vi "merFISH_set_autofocus_on_track.vi"(5 "queue ASI stage":refnum<queue>, 6 "error in":errorcluster, 7 "Slope":dbl, 8 "QPD ref":T1, 9 "queue piezo":refnum<queue>) -> (0 "error out":errorcluster)   [LabVIEW 2015]
uses:
  CONTROLS/Q_MCL_piezo_element.ctl
  CONTROLS/Q_ASI_stage_element.ctl
  <vilib>/Analysis/_algsub.llb/Vector Norm Type.ctl
  <vilib>/Analysis/_algsub.llb/Real Vector Norm.vi
  GLOBAL/Global_MCL_piezo.vi
  GLOBAL/Global_MAIN.vi
  GLOBAL/Global_FPGA.vi
  GLOBAL/Global_ABORT.vi
  <vilib>/regexp/Match Regular Expression.xnode
  <vilib>/Analysis/NI_AALPro.lvlib
panel:
  in  "abort":bool
  out "setpoint found":bool
  in  "resume":bool
  out "norm":dbl
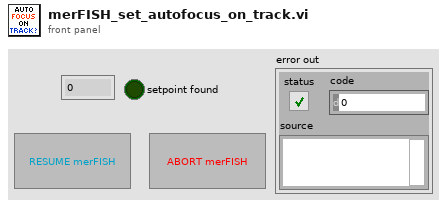
[diagram p1: front panel]
types:
  T1 = cluster{"X":sgl, "Y":sgl, "SUM":sgl, "count":u32}
  T2 = typedef "Q_MCL_piezo_element.ctl" = cluster{"variant":variant, "Instruction":enum16{"Piezo_idle", "Piezo_initialize", "Piezo_error", "Piezo_security_stop", "Piezo_read_z", "Piezo_move_z", "Piezo_keyboard_move", "Piezo_close_autofocus_calibration_ramp", "Piezo_change_init_state", "Piezo_init_autofocus", "Piezo_init_autofocus_merFISH_TL", "Piezo_autofocus", "Piezo_autofocus_merFISH_TL", "Piezo_stop_autofocus", "Piezo_stop_autofocus_merFISH_TL", "Piezo_autofocus_lost", "Piezo_resume_autofocus_merFISH_TL", "Piezo_check_z_position_merFISH_TL", "Piezo_init_ramp", "Piezo_move_z_ramp", "Piezo_close_ramp", "Piezo_close_merFISH", "Piezo_stop"}}
  T3 = typedef "NI_AALPro.lvlib/Vector Norm Type.ctl" = u16
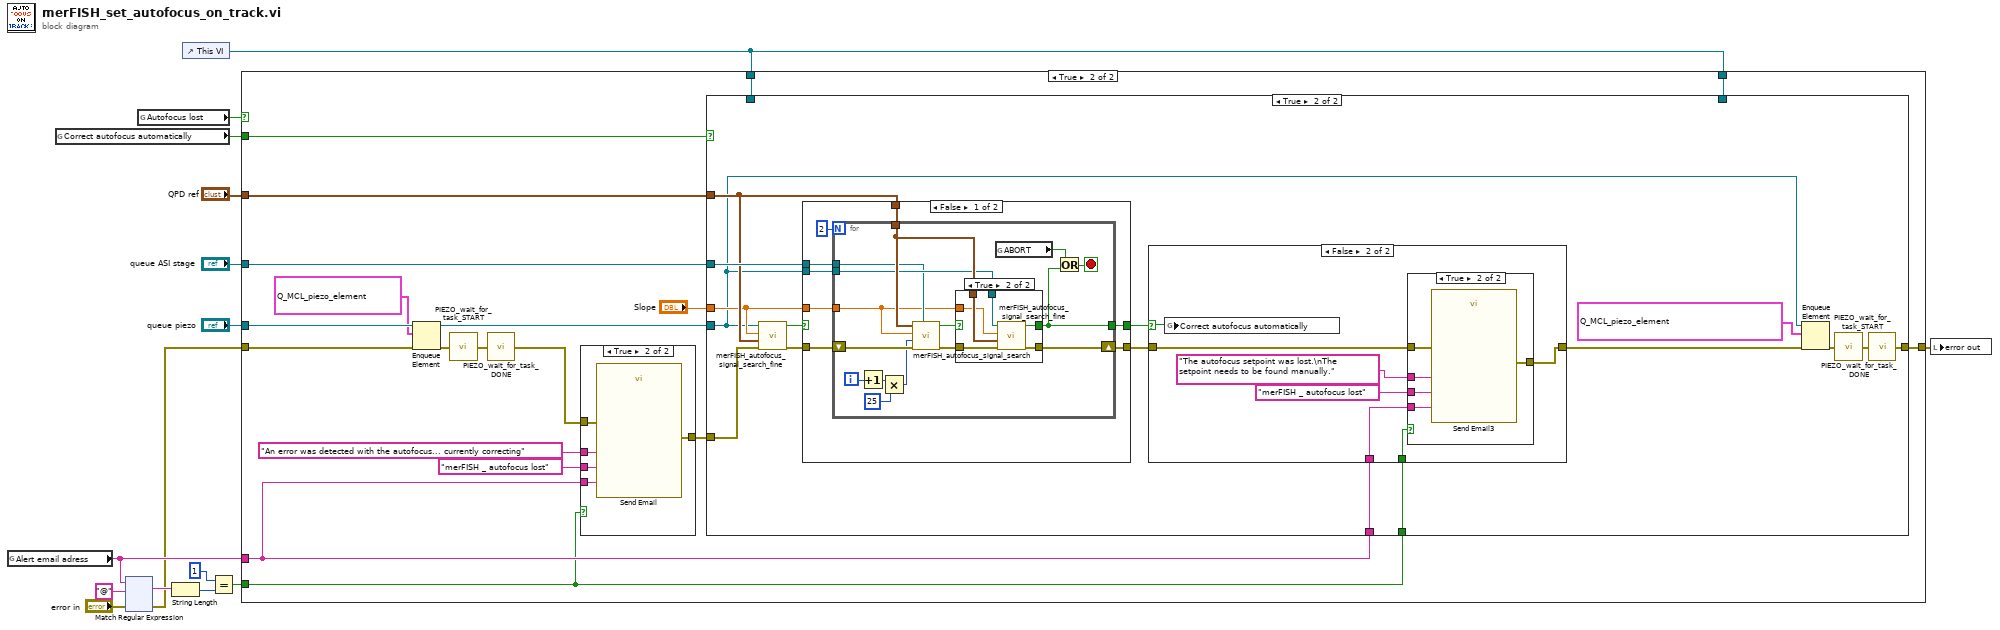
[diagram p0: block diagram]
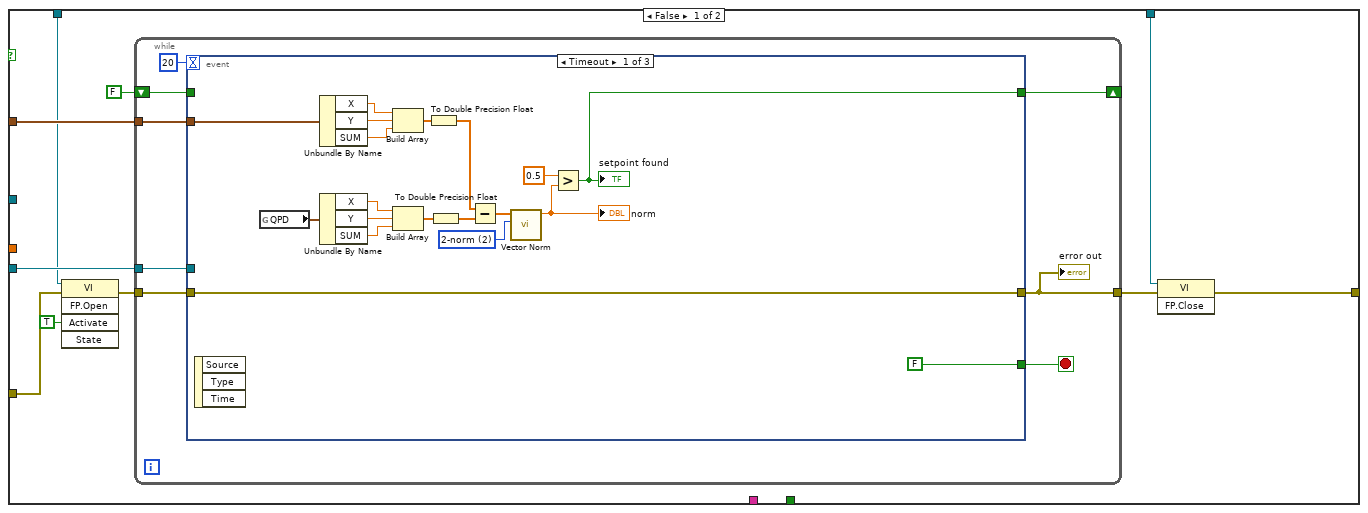
[diagram p4: hidden frame]
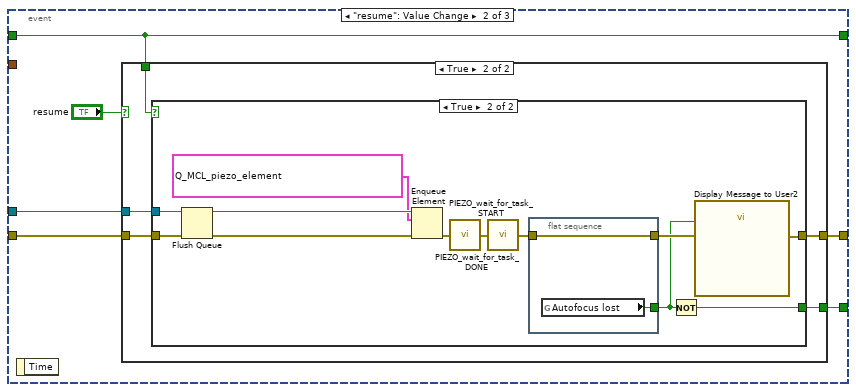
[diagram p5: hidden frame]
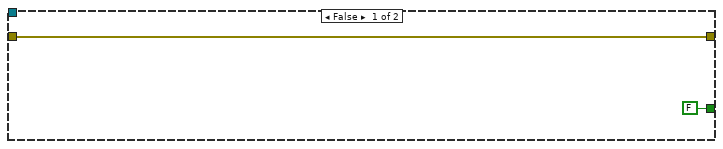
[diagram p6: hidden frame]
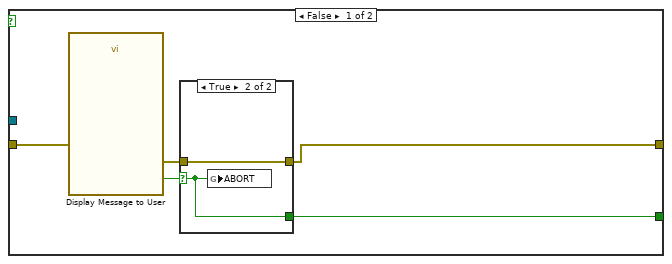
[diagram p7: hidden frame]
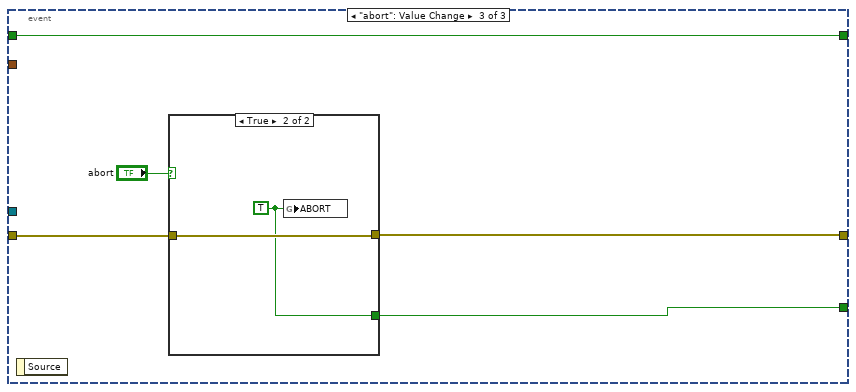
[diagram p9: hidden frame]
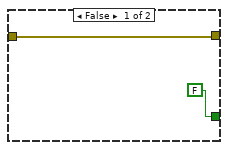
[diagram p10: hidden frame]
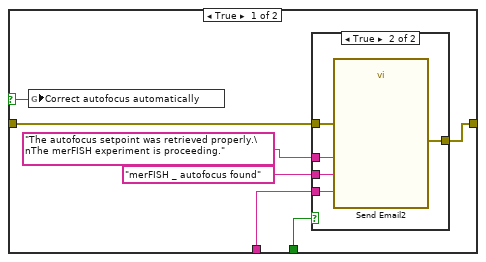
[diagram p13: hidden frame]
diagram:
  n1 = global read "Global_MAIN.vi" "Alert email adress"() -> (w5:string)
  n2 = global read "Global_MAIN.vi" "Correct autofocus automatically"() -> (w12:bool)
  n3 = xnode "Match Regular Expression"("input string"=w5, "regular expression"="@", "error in"="error in") -> ("whole match"=w7:string, "error out"=w3:errorcluster)  [unwired: 3 in, 3 out]
  n4 = global read "Global_MCL_piezo.vi" "Autofocus lost"() -> (w15:bool)
  n5 = String Length(string=w7) -> (length=w8:i32)
  n6 = control-ref of="This VI"() -> (w10:refnum<vi>)
  n7 = Equal?(x=1 ("y"), y=w8) -> (x = y?=w1:bool)
  n8 = case shown="True" w15 {
    tunnel: w3 -> [w16 w18]
    tunnel: "QPD ref" -> [_ w35]
    tunnel: "queue piezo" -> [_ w31]
    tunnel: [w16 w21] -> w13
    tunnel: w10 -> [_ w22]
    tunnel: w12 -> [_ w29]
    tunnel: "queue ASI stage" -> [_ w28]
    tunnel: w10 -> [_ w23]
    tunnel: w5 -> [_ w20]
    tunnel: w1 -> [_ w17]
    frame False {
    }
    frame True {
      n9 = Enqueue Element(queue=w31, element=T2 {"variant"=variant, "Instruction"=enum."Piezo_autofocus_lost"}, error in (no error)=w18) -> (queue out=w33:refnum<queue>, error out=w34:errorcluster)  [unwired: 1 in, 1 out]
      n10 = call "PIEZO_wait_for_task_START.vi"("error in"=w34) -> ("error out"=w32:errorcluster)
      n11 = call "PIEZO_wait_for_task_DONE.vi"("error in"=w32) -> ("error out"=w27:errorcluster)
      n12 = case shown="True" w17 {
        tunnel: w27 -> [w36 w41]
        tunnel: [w36 w40] -> w26
        tunnel: "merFISH _ autofocus lost" ("Subject") -> [_ w39]
        tunnel: "An error was detected with the autofocus... currently correcting" ("Message") -> [_ w38]
        tunnel: w20 -> [_ w37]
        frame False {
        }
        frame True {
          n13 = call "Send Email"("error in"=w41, "Message"=w38, "Subject"=w39, "Recipients"=w37) -> ("error out"=w40:errorcluster)  [unwired: 7 in]
        }
      }
      n14 = case shown="True" w29 {
        tunnel: w35 -> [w51 w129]
        tunnel: w33 -> [w50 w127]
        tunnel: w26 -> [w47 w130]
        tunnel: [w43 w131] -> w21
        tunnel: w28 -> [_ w139]
        tunnel: w23 -> [w45 _]
        tunnel: w22 -> [w42 _]
        tunnel: w20 -> [_ w137]
        tunnel: "Slope" -> [_ w128]
        tunnel: w17 -> [_ w124]
        frame False {
          n15 = invoke class="VI" method="FP.Open"(reference=w45, error in=w47, "Activate"=TRUE ("Activate?")) -> (error out=w46:errorcluster)  [unwired: 2 in, 4 out]
          n16 = while {
            tunnel: w46 -> [w59]
            tunnel: w51 -> [w58]
            tunnel: [w53] -> w44
            shift-right: [w56] -> _
            shift-left: FALSE -> [w55]
            tunnel: w50 -> [w52]
            stop <- w54 stop-if-true
            n17 = event shown="[0] Timeout" {
              selector: _ -> [_ _ _]
              dyn-events: _ -> [_ _ _]
              timeout: 20 -> [_ _ _]
              tunnel: w59 -> [w72 w84 w118]
              tunnel: w58 -> [w66 _ _]
              tunnel: [w72 w80 w117] -> w53
              tunnel: [w74 w83 w119] -> w56
              tunnel: w55 -> [_ w83 w119]
              tunnel: [FALSE ("resume") w79 w115] -> w54
              tunnel: w52 -> [_ w81 _]
              event Timeout {
                w77 = T3 2 items=["1-norm"=1, "2-norm"=2, "Inf-norm"=3, "-Inf-norm"=4, "User Defined"=5] ("norm type")
                n18 = event-data() -> ()  [unwired: 1 in, 3 out]
                n19 = global read "Global_FPGA.vi" "QPD"() -> (w71:T1)
                n20 = Unbundle By Name(w66) -> ("X"=w64:sgl, "Y"=w65:sgl, "SUM"=w63:sgl)
                n21 = Unbundle By Name(w71) -> ("X"=w69:sgl, "Y"=w70:sgl, "SUM"=w68:sgl)
                n22 = Build Array(w64, w65, w63) -> (w62:sgl[])
                n23 = Build Array(w69, w70, w68) -> (w67:sgl[])
                n24 = To Double Precision Float(number=w62) -> (double precision float=w61:dbl[])
                n25 = To Double Precision Float(number=w67) -> (double precision float=w60:dbl[])
                n26 = Subtract(x=w61, y=w60) -> (x-y=w78:dbl[])
                n27 = call-poly <vilib>:"Vector Norm.vi"("norm type"=w77, "Input Vector"=w78) -> ("norm"=w75:dbl)  [unwired: 8 in, 1 out]
                "norm" <- w75
                n28 = Greater?(x=0.5 ("y"), y=w75) -> (0:w74:bool)
                "setpoint found" <- w74
              }
              event "resume": Value Change {
                n29 = event-data() -> ()  [unwired: 1 in, 1 out]
                n30 = case shown="True" "resume" {
                  tunnel: w84 -> [w86 w91]
                  tunnel: [w86 w90] -> w80
                  tunnel: w83 -> [_ w89]
                  tunnel: w81 -> [_ w88]
                  tunnel: [FALSE w87] -> w79
                  frame False {
                  }
                  frame True {
                    n31 = case shown="True" w89 {
                      tunnel: w91 -> [w96 w112]
                      tunnel: [w93 w103] -> w90
                      tunnel: w88 -> [_ w106]
                      tunnel: [w92 w101] -> w87
                      frame False {
                        n32 = call "Display Message to User"("error in (no error)"=w96) -> ("error out"=w94:errorcluster, "Proceed"=w95:bool)  [unwired: 9 in]
                        n33 = case shown="True" w95 {
                          selector: w95 -> [w97 w99]
                          tunnel: w94 -> [w98 w100]
                          tunnel: [w98 w100] -> w93
                          tunnel: [w97 w99] -> w92
                          frame False {
                          }
                          frame True {
                            n34 = global write "Global_ABORT.vi" "ABORT"(w99) -> ()
                          }
                        }
                      }
                      frame True {
                        n35 = Flush Queue(queue=w106, error in (no error)=w112) -> (queue out=w110:refnum<queue>, error out=w111:errorcluster)  [unwired: 1 out]
                        n36 = Enqueue Element(queue=w110, element=T2 {"variant"=variant, "Instruction"=enum."Piezo_resume_autofocus_merFISH_TL"}, error in (no error)=w111) -> (error out=w108:errorcluster)  [unwired: 1 in, 2 out]
                        n37 = call "PIEZO_wait_for_task_START.vi"("error in"=w108) -> ("error out"=w107:errorcluster)
                        n38 = call "PIEZO_wait_for_task_DONE.vi"("error in"=w107) -> ("error out"=w105:errorcluster)
                        n39 = flat-sequence {
                          tunnel: w105 -> [w114]
                          tunnel: [w114] -> w104
                          tunnel: [w113] -> w102
                          frame #0 {
                            n40 = global read "Global_MCL_piezo.vi" "Autofocus lost"() -> (w113:bool)
                          }
                        }
                        n41 = Not(x=w102) -> (.not. x?=w101:bool)
                        n42 = call "Display Message to User2"("error in (no error)"=w104, "Enable"=w102) -> ("error out"=w103:errorcluster)  [unwired: 8 in, 1 out]
                      }
                    }
                  }
                }
              }
              event "abort": Value Change {
                n43 = event-data() -> ()  [unwired: 1 in, 1 out]
                n44 = case shown="True" "abort" {
                  tunnel: [w121 w123] -> w117
                  tunnel: w118 -> [w121 w123]
                  tunnel: [FALSE ("ABORT") w122] -> w115
                  frame False {
                  }
                  frame True {
                    w122 = TRUE ("ABORT")
                    n45 = global write "Global_ABORT.vi" "ABORT"(w122) -> ()
                  }
                }
              }
            }
            "error out" <- w53
          }
          n46 = invoke class="VI" method="FP.Close"(reference=w42, error in=w44) -> (error out=w43:errorcluster)  [unwired: 1 in, 2 out]
        }
        frame True {
          n47 = call "merFISH_autofocus_signal_search_fine.vi"("error in"=w130, "QPD ref"=w129, "Slope"=w128, "queue piezo"=w127) -> ("error out"=w126:errorcluster, "Ref found?"=w125:bool)  [unwired: 3 in]
          n48 = case shown="False" w125 {
            selector: w125 -> [_ w171]
            tunnel: w139 -> [w146 _]
            tunnel: [w145 w172] -> w138
            tunnel: [w144 w171] -> w136
            tunnel: w129 -> [w143 _]
            tunnel: w128 -> [w142 _]
            tunnel: w127 -> [w141 _]
            tunnel: w126 -> [w140 w172]
            frame False {
              n49 = for {
                N: 2 -> [_]
                tunnel: w143 -> [w160]
                shift-right: [w159] -> w145
                shift-left: w140 -> [w162]
                tunnel: w141 -> [w152]
                tunnel: w146 -> [w151]
                tunnel: [w150] -> w144
                tunnel: w142 -> [w148]
                i -> [w158]
                stop <- w154 stop-if-true
                n50 = Increment(x=w158) -> (x+1=w157:i32)
                n51 = Multiply(x=w157, y=25) -> (x*y=w155:i32)
                n52 = call "merFISH_autofocus_signal_search.vi"("queue ASI stage"=w151, "error in"=w162, "Search range"=w155, "Slope"=w148, "QPD ref"=w160) -> ("error out"=w161:errorcluster, "Ref found?"=w149:bool)  [unwired: 3 in]
                n53 = case shown="True" w149 {
                  selector: w149 -> [w163 _]
                  tunnel: w161 -> [w164 w170]
                  tunnel: w160 -> [_ w169]
                  tunnel: [w164 w168] -> w159
                  tunnel: w152 -> [_ w167]
                  tunnel: [w163 w166] -> w150
                  tunnel: w148 -> [_ w165]
                  frame False {
                  }
                  frame True {
                    n54 = call "merFISH_autofocus_signal_search_fine.vi"("error in"=w170, "QPD ref"=w169, "Slope"=w165, "queue piezo"=w167) -> ("error out"=w168:errorcluster, "Ref found?"=w166:bool)  [unwired: 3 in]
                  }
                }
                n55 = global read "Global_ABORT.vi" "ABORT"() -> (w153:bool)
                n56 = Or(x=w153, y=w150) -> (x .or. y?=w154:bool)
              }
            }
            frame True {
            }
          }
          n57 = case shown="False" w136 {
            selector: w136 -> [w174 w187]
            tunnel: w138 -> [w179 w192]
            tunnel: [w178 w191] -> w135
            tunnel: w137 -> [w177 w190]
            tunnel: w124 -> [w173 w186]
            frame True {
              n58 = global write "Global_MAIN.vi" "Correct autofocus automatically"(w174) -> ()
              n59 = case shown="True" w173 {
                tunnel: w179 -> [w180 w185]
                tunnel: [w180 w184] -> w178
                tunnel: w177 -> [_ w183]
                tunnel: "merFISH _ autofocus found" ("Subject") -> [_ w182]
                tunnel: "The autofocus setpoint was retrieved properly.\nThe merFISH experiment is proceeding." ("Message") -> [_ w181]
                frame False {
                }
                frame True {
                  n60 = call "Send Email2"("error in"=w185, "Message"=w181, "Subject"=w182, "Recipients"=w183) -> ("error out"=w184:errorcluster)  [unwired: 7 in]
                }
              }
            }
            frame False {
              n61 = global write "Global_MAIN.vi" "Correct autofocus automatically"(w187) -> ()
              n62 = case shown="True" w186 {
                tunnel: w192 -> [w193 w198]
                tunnel: [w193 w197] -> w191
                tunnel: w190 -> [_ w196]
                tunnel: "merFISH _ autofocus lost" ("Subject") -> [_ w195]
                tunnel: "The autofocus setpoint was lost.\nThe setpoint needs to be found manually." ("Message") -> [_ w194]
                frame False {
                }
                frame True {
                  n63 = call "Send Email3"("error in"=w198, "Message"=w194, "Subject"=w195, "Recipients"=w196) -> ("error out"=w197:errorcluster)  [unwired: 7 in]
                }
              }
            }
          }
          n64 = Enqueue Element(queue=w127, element=T2 {"variant"=variant, "Instruction"=enum."Piezo_resume_autofocus_merFISH_TL"}, error in (no error)=w135) -> (error out=w133:errorcluster)  [unwired: 1 in, 2 out]
          n65 = call "PIEZO_wait_for_task_START.vi"("error in"=w133) -> ("error out"=w132:errorcluster)
          n66 = call "PIEZO_wait_for_task_DONE.vi"("error in"=w132) -> ("error out"=w131:errorcluster)
        }
      }
    }
  }
  n67 = local write "error out"(w13) -> ()
